vi "LV Exp9.vi"() -> ()   [LabVIEW 2009]
uses:
  <vilib>/NXT/Block Support/NXT_InputPort.ctl
  <vilib>/NXT/Dual Mode Library/Waits/Wait_Num(msec).vi
panel:
  in  "Analog Mode":u8(ring)=2 items=["DC", "Sine Wave", "Square Wave", "Pos Sawtooth Wave", "Neg Sawtooth Wave", "Triangle Wave", "PWM Voltage"]
  # "HiTechnic Experimenter's Kit\n\n                        Experiment 9 - Speaker\nThis program  first plays a sequence of three ascending\nnotes using just O0 and then three pairs of descending\nnotes using both O0 and O1.\n\nSee Experimenter's Kit Handbook for the SuperPro for\nmore information or go to www.hitechnic.com.\n\n(c) HiTechnic 2011"
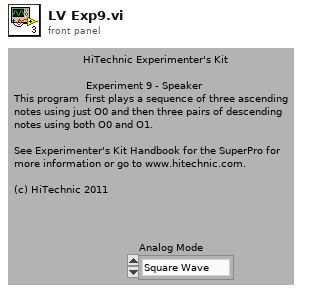
[diagram p1: front panel]
types:
  T1 = typedef "NXT_InputPort.ctl" = u8
  T2 = typedef "LVHSConnector.ctl" = cluster{"error":errorcluster, "address":string, "NXT #":i32, "Show Error":bool, "Connection":u16}
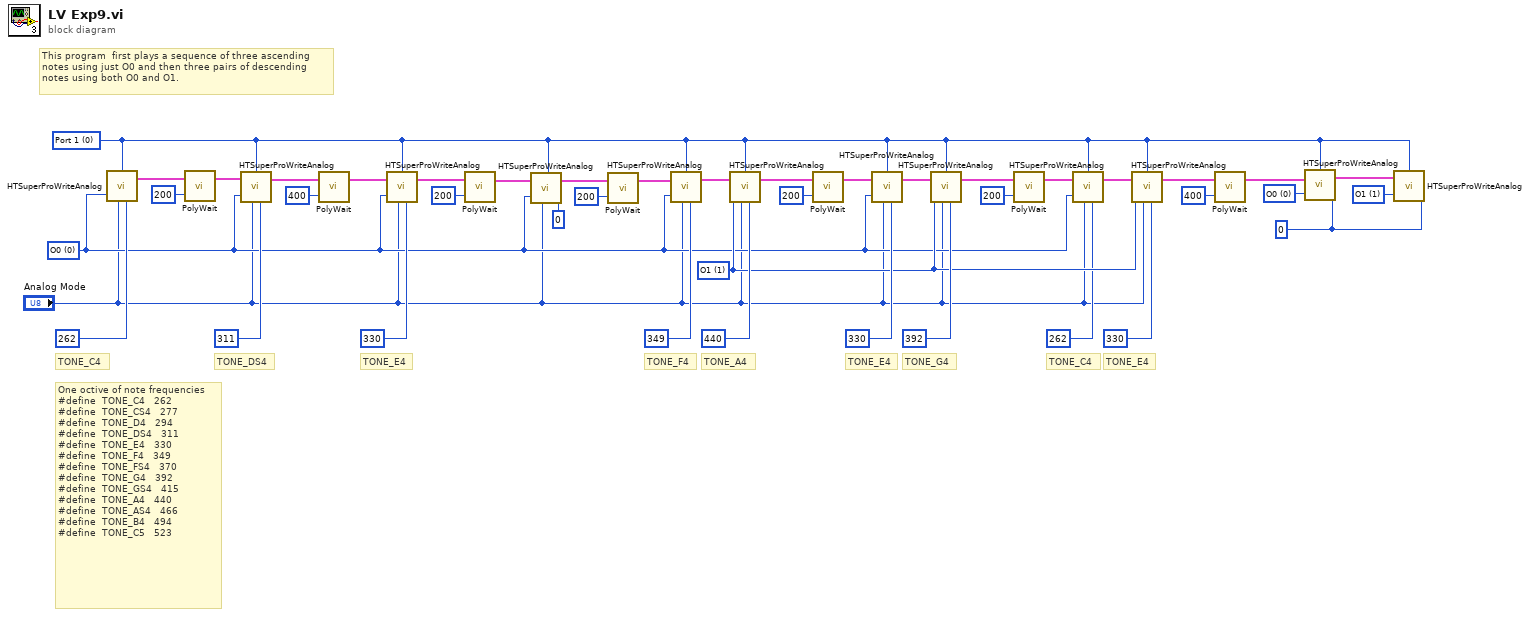
[diagram p0: block diagram]
diagram:
  w12 = u8 1 items=["O0", "O1"] ("Analog Output")
  w38 = u8 1 items=["O0", "O1"] ("AnalogOutput")
  w39 = u8 0 items=["O0", "O1"] ("AnalogOutput")
  w40 = i16 0 ("Voltage")
  w11 = u8 0 items=["O0", "O1"] ("AnalogOutput")
  w8 = T1 0 items=["Port 1", "Port 2", "Port 3", "Port 4"] ("Port")
  # "One octive of note frequencies\n#define  TONE_C4   262 \n#define  TONE_CS4   277 \n#define  TONE_D4   294 \n#define  TONE_DS4   311 \n#define  TONE_E4   330 \n#define  TONE_F4   349 \n#define  TONE_FS4   370 \n#define  TONE_G4   392 \n#define  TONE_GS4   415 \n#define  TONE_A4   440 \n#define  TONE_AS4   466 \n#define  TONE_B4   494 \n#define  TONE_C5   523"
  # "This program  first plays a sequence of three ascending\nnotes using just O0 and then three pairs of descending\nnotes using both O0 and O1."
  # "TONE_E4"
  # "TONE_C4"
  # "TONE_G4"
  # "TONE_E4"
  # "TONE_A4"
  # "TONE_F4"
  # "TONE_E4"
  # "TONE_DS4"
  # "TONE_C4"
  n1 = call "HTSuperProWriteAnalog.vi"("Port"=w8, "Frequency"=i16 262, "Analog Mode"="Analog Mode", "Analog Output"=w11) -> ("NXT"=w28:T2)  [unwired: 2 in]
  n2 = call-poly <vilib>:"PolyWait.vi"("Time (msec)"=u32 200 ("Time (100 msec)"), "NXT"=w28) -> ("NXT"=w27:T2)  [unwired: 2 in]
  n3 = call "HTSuperProWriteAnalog.vi"("Port"=w8, "NXT"=w27, "Frequency"=i16 311, "Analog Mode"="Analog Mode", "Analog Output"=w11) -> ("NXT"=w26:T2)  [unwired: 1 in]
  n4 = call-poly <vilib>:"PolyWait.vi"("Time (msec)"=u32 400 ("Time (100 msec)"), "NXT"=w26) -> ("NXT"=w25:T2)  [unwired: 2 in]
  n5 = call "HTSuperProWriteAnalog.vi"("Port"=w8, "NXT"=w25, "Frequency"=i16 330, "Analog Mode"="Analog Mode", "Analog Output"=w11) -> ("NXT"=w33:T2)  [unwired: 1 in]
  n6 = call-poly <vilib>:"PolyWait.vi"("Time (msec)"=u32 200 ("Time (100 msec)"), "NXT"=w33) -> ("NXT"=w31:T2)  [unwired: 2 in]
  n7 = call "HTSuperProWriteAnalog.vi"("Port"=w8, "NXT"=w31, "Voltage"=i16 0, "Analog Mode"="Analog Mode", "Analog Output"=w11) -> ("NXT"=w7:T2)  [unwired: 1 in]
  n8 = call-poly <vilib>:"PolyWait.vi"("Time (msec)"=u32 200 ("Time (100 msec)"), "NXT"=w7) -> ("NXT"=w6:T2)  [unwired: 2 in]
  n9 = call "HTSuperProWriteAnalog.vi"("Port"=w8, "NXT"=w6, "Frequency"=i16 349, "Analog Mode"="Analog Mode", "Analog Output"=w11) -> ("NXT"=w5:T2)  [unwired: 1 in]
  n10 = call "HTSuperProWriteAnalog.vi"("Port"=w8, "NXT"=w5, "Frequency"=i16 440, "Analog Mode"="Analog Mode", "Analog Output"=w12) -> ("NXT"=w4:T2)  [unwired: 1 in]
  n11 = call-poly <vilib>:"PolyWait.vi"("Time (msec)"=u32 200 ("Time (100 msec)"), "NXT"=w4) -> ("NXT"=w3:T2)  [unwired: 2 in]
  n12 = call "HTSuperProWriteAnalog.vi"("Port"=w8, "NXT"=w3, "Frequency"=i16 330, "Analog Mode"="Analog Mode", "Analog Output"=w11) -> ("NXT"=w20:T2)  [unwired: 1 in]
  n13 = call "HTSuperProWriteAnalog.vi"("Port"=w8, "NXT"=w20, "Frequency"=i16 392, "Analog Mode"="Analog Mode", "Analog Output"=w12) -> ("NXT"=w2:T2)  [unwired: 1 in]
  n14 = call-poly <vilib>:"PolyWait.vi"("Time (msec)"=u32 200 ("Time (100 msec)"), "NXT"=w2) -> ("NXT"=w14:T2)  [unwired: 2 in]
  n15 = call "HTSuperProWriteAnalog.vi"("Port"=w8, "NXT"=w14, "Frequency"=i16 262, "Analog Mode"="Analog Mode", "Analog Output"=w11) -> ("NXT"=w16:T2)  [unwired: 1 in]
  n16 = call "HTSuperProWriteAnalog.vi"("Port"=w8, "NXT"=w16, "Frequency"=i16 330, "Analog Mode"="Analog Mode", "Analog Output"=w12) -> ("NXT"=w13:T2)  [unwired: 1 in]
  n17 = call-poly <vilib>:"PolyWait.vi"("Time (msec)"=u32 400 ("Time (100 msec)"), "NXT"=w13) -> ("NXT"=w9:T2)  [unwired: 2 in]
  n18 = call "HTSuperProWriteAnalog.vi"("Port"=w8, "NXT"=w9, "Voltage"=w40, "Analog Output"=w39) -> ("NXT"=w41:T2)  [unwired: 2 in]
  n19 = call "HTSuperProWriteAnalog.vi"("Port"=w8, "NXT"=w41, "Voltage"=w40, "Analog Output"=w38) -> ()  [unwired: 2 in, 1 out]
